vi "质控单元全局.vi"() -> ()   [LabVIEW 2016]
panel:
  in  "状态":T1
  in  "启动记录":string
  in  "启动模式":u16
  in  "质控单元串口参数":T2={"VISA resource name"="", "baud rate (设置)"=115200, "unit ID"=1}
  out "启动运行次数":i32
  out "流程运行中":bool
  out "启动命令（模式）":string="空闲"
  out "运行状态":string
  in  "步骤时间/秒":T3={"步骤1时间"=2, "步骤2时间"=4, "步骤3时间"=2, "步骤4时间"=5, "步骤5时间"=6, "步骤6时间"=3, "步骤7时间"=4, "步骤8时间"=7, "步骤9时间"=8, "步骤10时间"=6}
  out "当前步骤":T4(ring)
  out "步骤运行时间/秒":i32
  out "流程结束":bool
  # "流程"
  # "流程步骤"
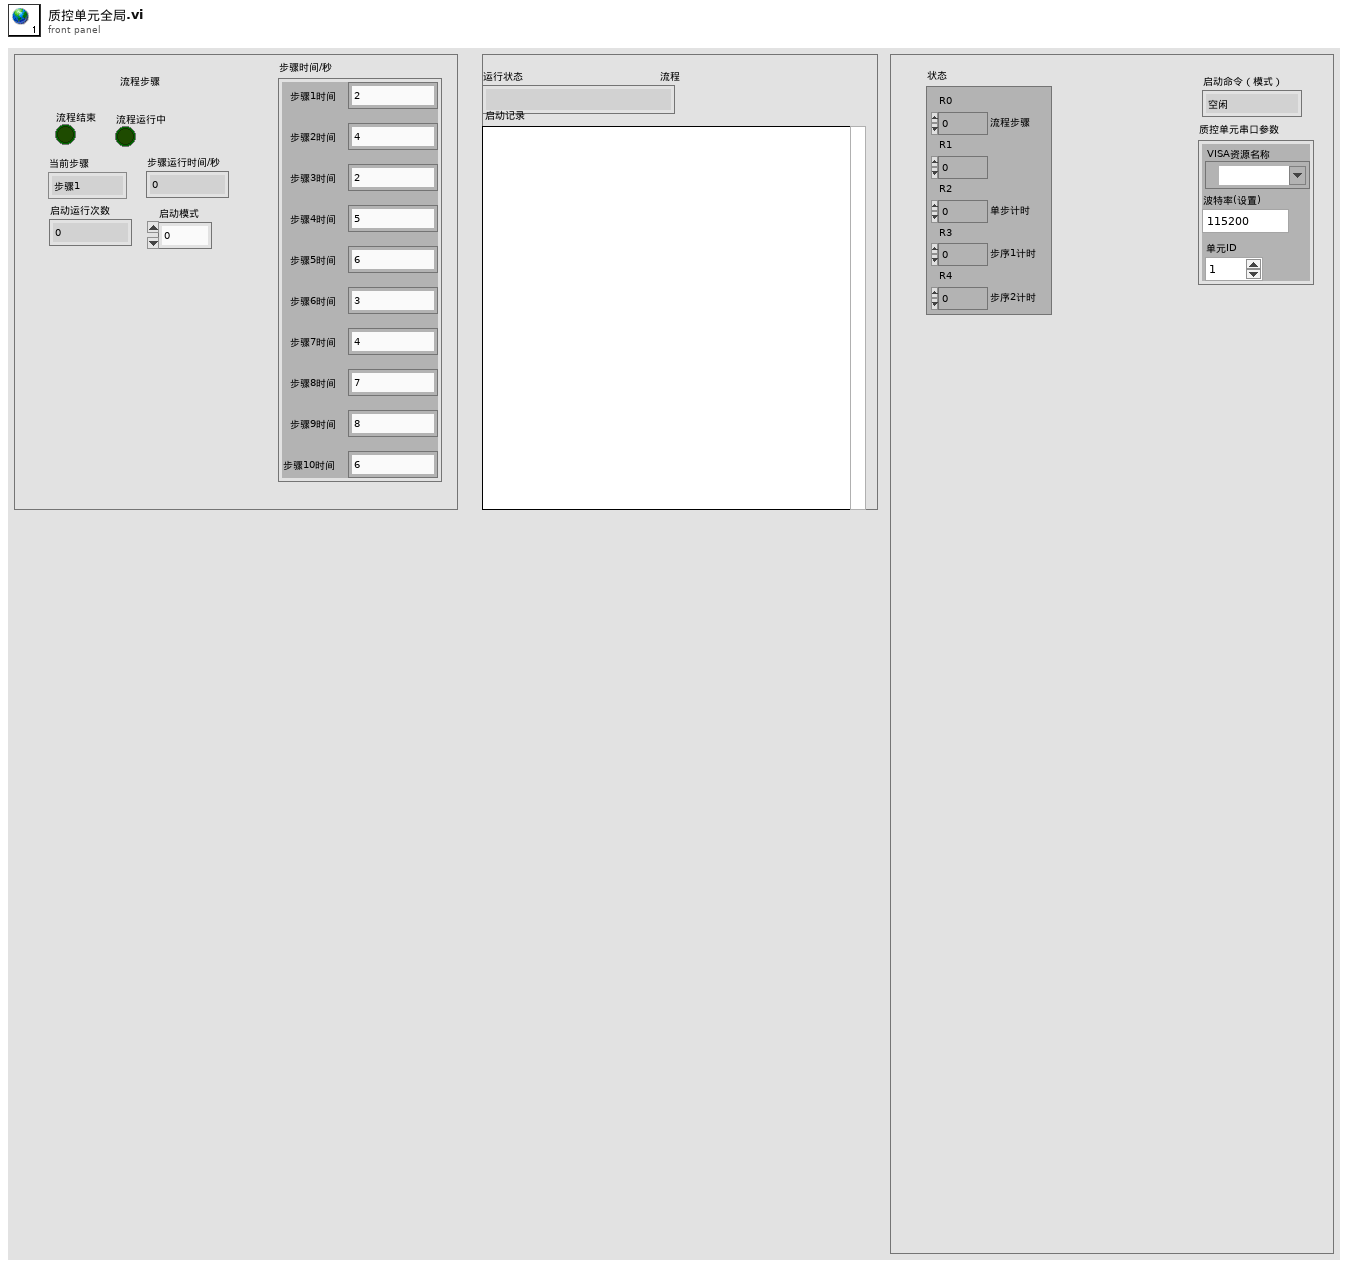
[diagram p1: front panel]
types:
  T1 = cluster{"R0":i16, "R1":i16, "R2":i16, "R3":i16, "R4":i16}
  T2 = cluster{"VISA resource name":refnum<visa-resource-name>, "baud rate (设置)":u32, "unit ID":u8}
  T3 = cluster{"步骤1时间":i32, "步骤2时间":i32, "步骤3时间":i32, "步骤4时间":i32, "步骤5时间":i32, "步骤6时间":i32, "步骤7时间":i32, "步骤8时间":i32, "步骤9时间":i32, "步骤10时间":i32}
  T4 = enum16{"步骤1", "步骤2", "步骤3", "步骤4", "步骤5", "步骤6", "步骤7", "步骤8", "步骤9", "步骤10"}
diagram:
